vi "Config Transmissores.vi"(6 "conversao corrente":bool, 8 "MAX":i32, 9 "MIN":i32, 10 "Corrente(mA)":dbl, 11 "tensão":dbl) -> (3 "valor":dbl)   [LabVIEW 2019]
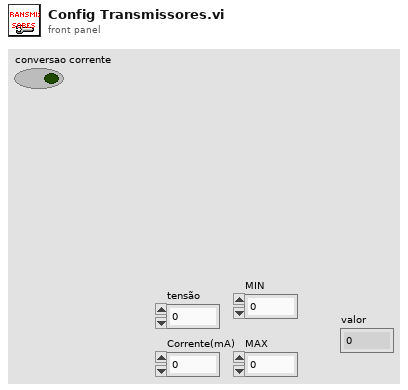
[diagram p1: front panel]
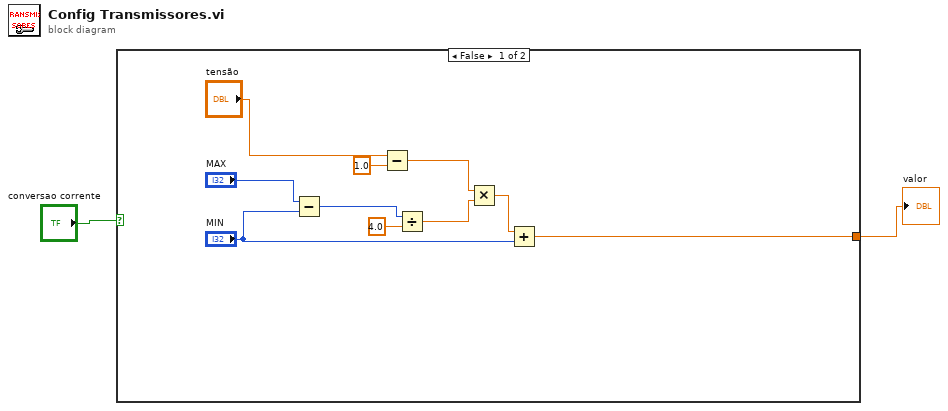
[diagram p0: block diagram]
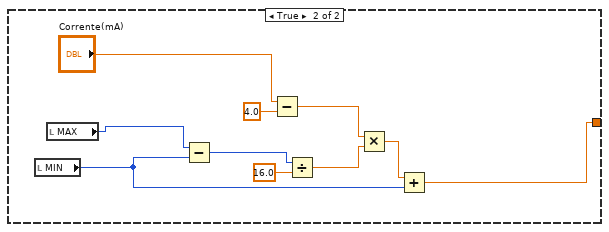
[diagram p2: hidden frame]
diagram:
  n1 = case shown="False" "conversao corrente" {
    tunnel: [w3 w16] -> w2
    frame False {
      n2 = Subtract(x="MAX", y="MIN") -> (x-y=w11:i32)
      n3 = Subtract(x="tensão", y=1.0) -> (x-y=w7:dbl)
      n4 = Divide(x=w11, y=4.0) -> (x/y=w6:dbl)
      n5 = Multiply(x=w7, y=w6) -> (x*y=w5:dbl)
      n6 = Add(x=w5, y="MIN") -> (x+y=w3:dbl)
    }
    frame True {
      n7 = local read "MIN"() -> (w15:i32)
      n8 = local read "MAX"() -> (w14:i32)
      n9 = Subtract(x=w14, y=w15) -> (x-y=w22:i32)
      n10 = Subtract(x="Corrente(mA)", y=4.0) -> (x-y=w19:dbl)
      n11 = Divide(x=w22, y=16.0) -> (x/y=w18:dbl)
      n12 = Multiply(x=w19, y=w18) -> (x*y=w17:dbl)
      n13 = Add(x=w17, y=w15) -> (x+y=w16:dbl)
    }
  }
  "valor" <- w2
